vi "MultiLineString_GOOPKernel.vi"(0 "Ref in":i32, 1 "Data in":T4, 2 "Data shared in":T2, 3 "VI ref":string, 4 "Dynamic VI path":path, 5 "Subclass folders":path[](array[path]), 6 "Subclass names":string[](array[string]), 7 "error in (no error)":errorcluster, 8 "Action":T3, 9 "Subclass?":bool, 10 "Object name":string, 11 "Dynamic VI name":string, 13 "First try?":bool, 15 "Occurrence":refnum<k4>, 17 "Occurrence shared":refnum<k4>) -> (14 "Occurrence out":refnum<k4>, 16 "# of objects":i32, 18 "Class statistics":T1, 19 "IsSubclass?":bool, 20 "Ref out":i32, 21 "Data out":T4, 22 "Data shared out":T2, 23 "VI ref out":string, 24 "Dynamic VI path out":path, 25 "Exists?":bool, 26 "Data locked?":bool, 27 "error out":errorcluster)   [LabVIEW 2012, in "MultiLineString.lvclass"]
doc: "This VIs manages objects of the MultiLineString.\n\n[GOOP 2.0.15]"
uses:
  <resource>/Framework/Providers/Open_GDS/UML/MultiLineString_class/MultiLineString.lvclass
  <resource>/Framework/Providers/Open_GDS/UML/MultiLineString_class/protected/ObjectAttributes.ctl
  <resource>/Framework/Providers/Open_GDS/UML/MultiLineString_class/JustificationType.ctl
  <resource>/Framework/Providers/Open_GDS/UML/MultiLineString_class/SizeType.ctl
  <vilib>/addons/_goop3.llb/3GOOPStates.ctl
  <resource>/Framework/Providers/Open_GDS/UML/MultiLineString_class/protected/ClassAttributes.ctl
  <vilib>/addons/_goop3.llb/3GOOPClassStatistics.ctl
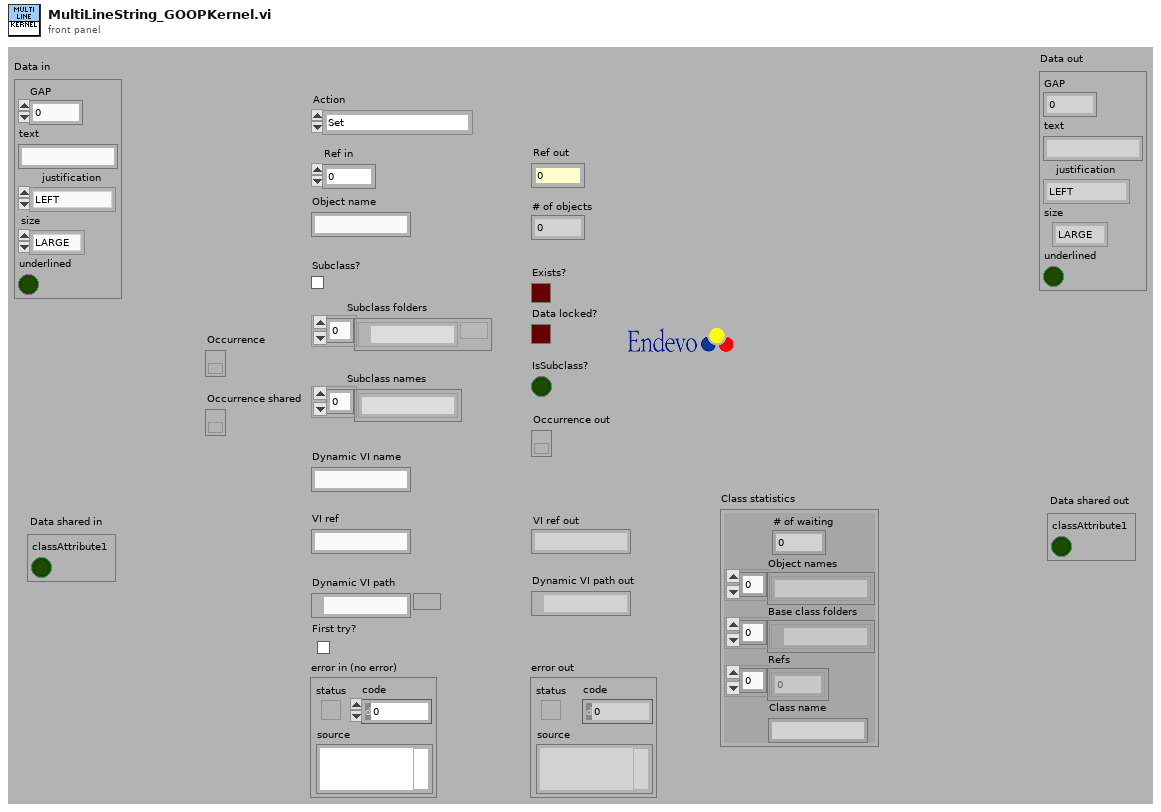
[diagram p1: front panel]
types:
  T1 = typedef "3GOOPClassStatistics.ctl" = cluster{"# of waiting":u32, "Object names":string[], "Base class folders":path[], "Refs":i32[], "Class name":string}
  T2 = typedef "MultiLineString.lvclass/ClassAttributes.ctl" = cluster{"classAttribute1":bool}
  T3 = typedef "3GOOPStates.ctl" = enum16{"Set", "Get", "New", "Delete", "Clear", "Test and get", "Unlock data", "Information", "Look up existing", "New or look up existing", "Test and get shared", "Get shared", "Set shared", "Unlock shared", "Find dynamic method", "Register dynamic method", "Preload dynamic method", "Probe", "Cast to more generic", "Cast to more specific"}
  T4 = typedef "MultiLineString.lvclass/ObjectAttributes.ctl" = cluster{"GAP":i32, "text":string, "justification":T5, "size":T6, "underlined":bool}
  T5 = typedef "MultiLineString.lvclass/JustificationType.ctl" = enum16{"LEFT", "CENTER", "RIGHT"}
  T6 = typedef "MultiLineString.lvclass/SizeType.ctl" = enum16{"LARGE", "NORMAL", "SMALL"}
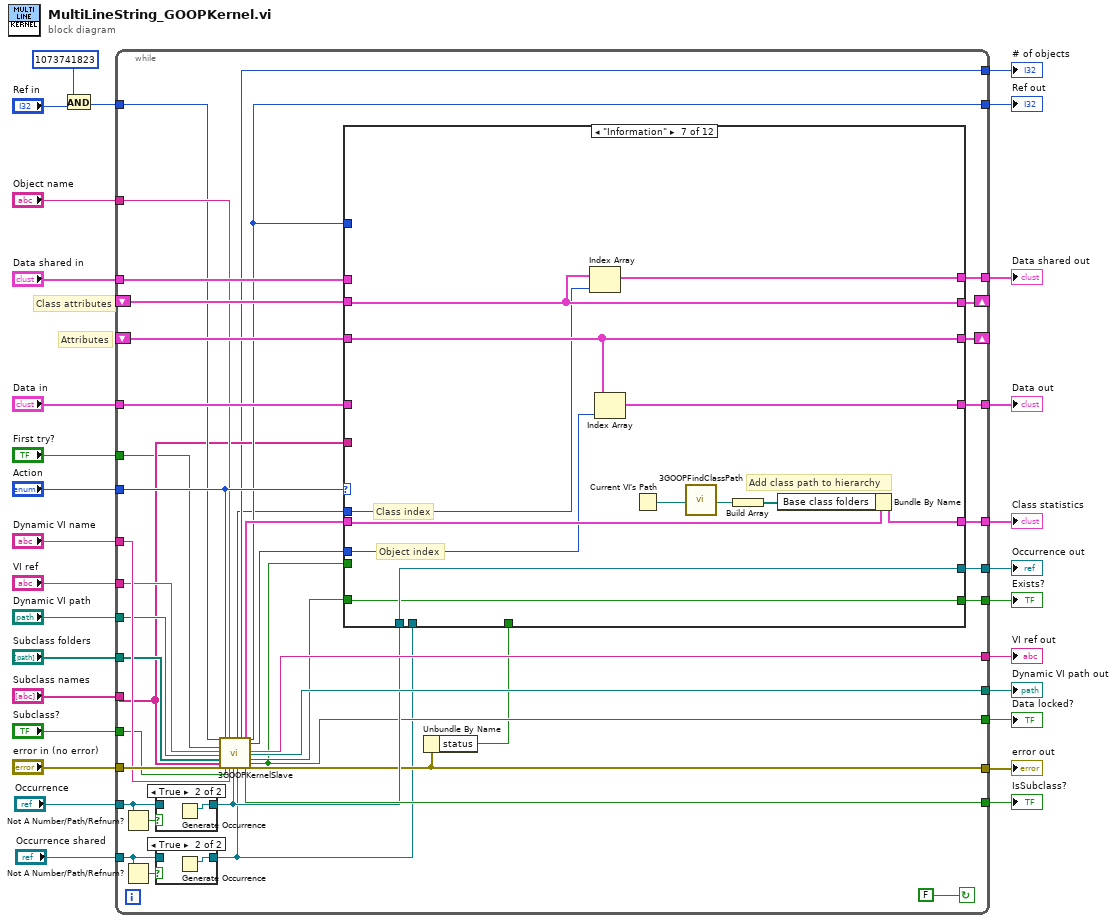
[diagram p0: block diagram]
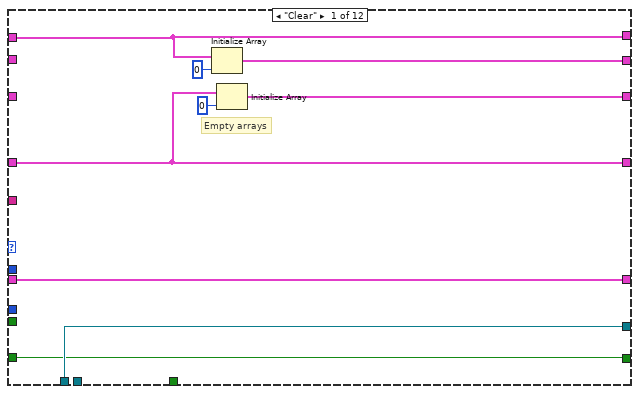
[diagram p4: hidden frame]
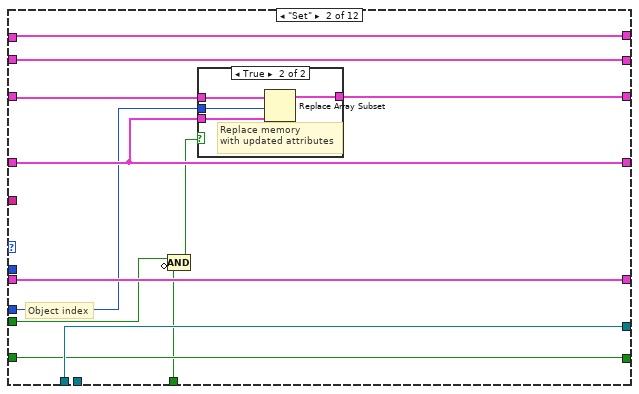
[diagram p5: hidden frame]
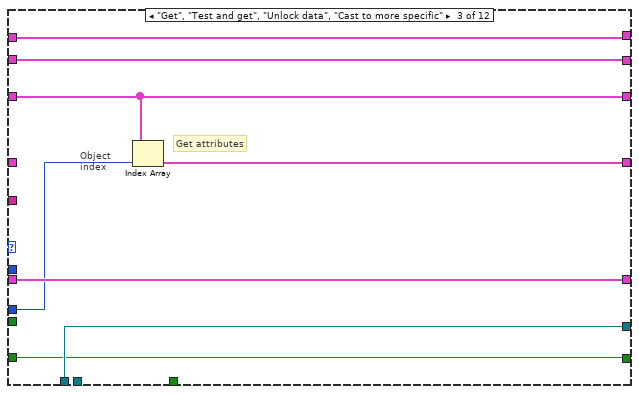
[diagram p7: hidden frame]
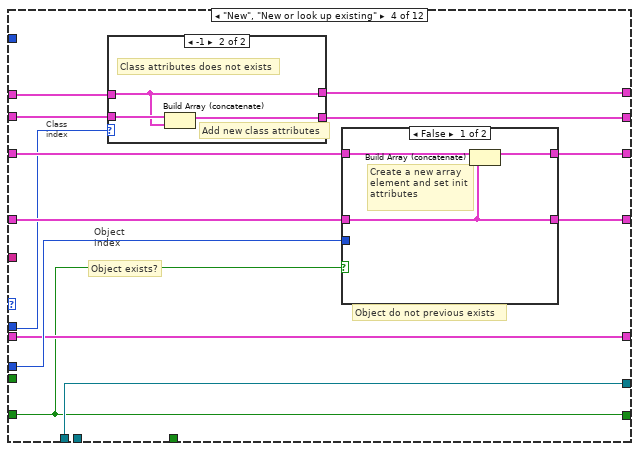
[diagram p8: hidden frame]
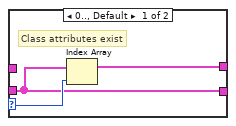
[diagram p9: hidden frame]
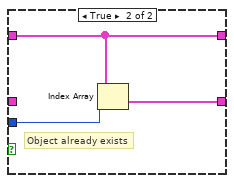
[diagram p10: hidden frame]
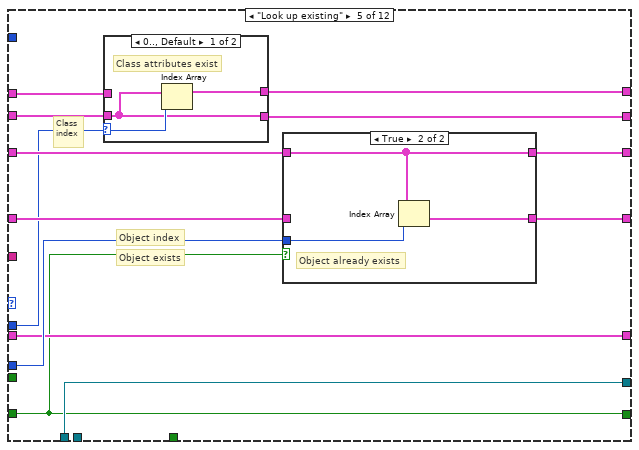
[diagram p11: hidden frame]
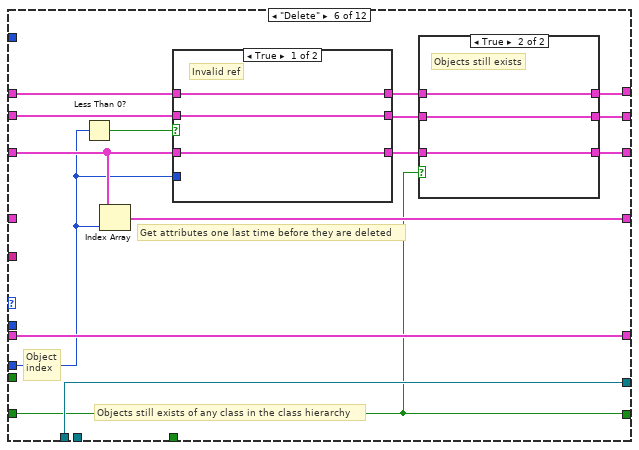
[diagram p14: hidden frame]
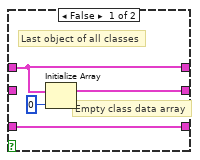
[diagram p15: hidden frame]
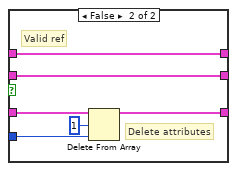
[diagram p16: hidden frame]
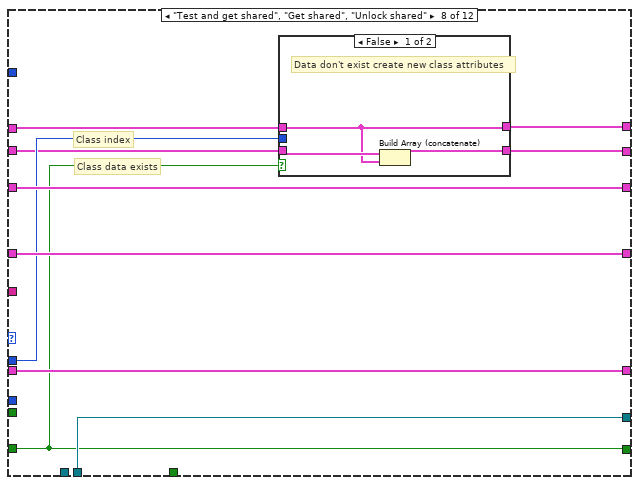
[diagram p17: hidden frame]
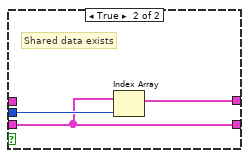
[diagram p18: hidden frame]
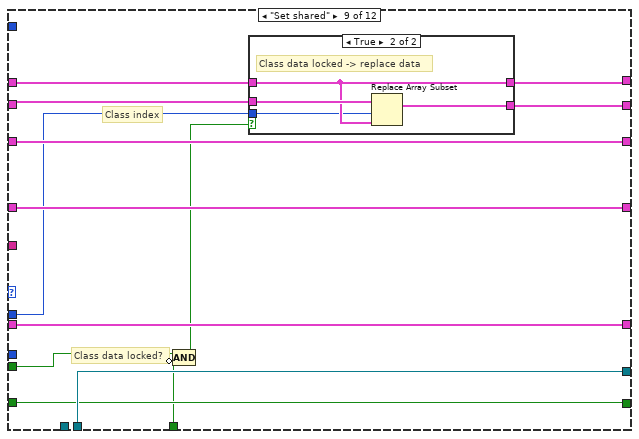
[diagram p19: hidden frame]
diagram:
  # "Attributes"
  # "Class attributes"
  n1 = And(x=1073741823 ("x .and. y?"), y="Ref in") -> (x .and. y?=w3:i32)
  n2 = while {
    tunnel: [w37] -> w6
    tunnel: [w41] -> w7
    tunnel: [w43] -> w8
    tunnel: "First try?" -> [w44]
    tunnel: [w46] -> w10
    tunnel: [w47] -> w11
    tunnel: [w62] -> w13
    tunnel: "Subclass folders" -> [w58]
    tunnel: "Subclass names" -> [w45]
    tunnel: "VI ref" -> [w56]
    tunnel: [w51] -> w17
    tunnel: "Dynamic VI path" -> [w57]
    tunnel: [w50] -> w19
    tunnel: "Dynamic VI name" -> [w60]
    tunnel: "Data shared in" -> [w63]
    shift-left: _ -> [w64]
    shift-right: [w65] -> _
    tunnel: "Object name" -> [w54]
    tunnel: [w36] -> w23
    tunnel: "error in (no error)" -> [w61]
    tunnel: "Subclass?" -> [w59]
    tunnel: [w38] -> w26
    tunnel: [w48] -> w27
    tunnel: w3 -> [w49]
    shift-left: _ -> [w68]
    shift-right: [w69] -> _
    tunnel: [w70] -> w28
    tunnel: "Action" -> [w55]
    tunnel: "Data in" -> [w67]
    tunnel: "Occurrence shared" -> [w33]
    tunnel: "Occurrence" -> [w30]
    stop <- FALSE continue-if-true
    n3 = Not A Number/Path/Refnum?(number/path/refnum=w30) -> (NaN/Path/Refnum?=w31:bool)
    n4 = Not A Number/Path/Refnum?(number/path/refnum=w33) -> (NaN/Path/Refnum?=w34:bool)
    n5 = case shown="True" w31 {
      tunnel: w30 -> [w71 _]
      tunnel: [w71 w72] -> w42
      frame False {
      }
      frame True {
        n6 = Generate Occurrence() -> (w72:refnum<k4>)
      }
    }
    n7 = case shown="True" w34 {
      tunnel: w33 -> [w73 _]
      tunnel: [w73 w74] -> w32
      frame False {
      }
      frame True {
        n8 = Generate Occurrence() -> (w74:refnum<k4>)
      }
    }
    n9 = call <vilib>:"3GOOPKernelSlave.vi"("ref in"=w49, "Misc"=w44, "Probe in"=w56, "Dynamic VI path"=w57, "Subclass folders"=w58, "Subclass names"=w45, "error in (no error)"=w61, "Action"=w55, "Subclass?"=w59, "Object name"=w54, "Class name"=w60, "Occurrence"=w42, "Occurrence shared"=w32) -> ("Shared index out"=w40:i32, "# of objects"=w43:i32, "Class statistics"=w52:T1, "IsSubclass?"=w47:bool, "ref out"=w48:i32, "Index out"=w53:i32, "Probe out"=w50:string, "Dynamic VI path out"=w51:path, "Exists/DynamicCall?"=w39:bool, "Data locked?"=w38:bool, "error out"=w36:errorcluster)  [unwired: 1 in, 3 out]
    n10 = Unbundle By Name(w36) -> ("status"=w35:bool)
    n11 = case shown="\"Information\"" w55 {
      tunnel: [w77 w95 w107 w118 w143 w168 w199 w210 w228 w242 w253 w254] -> w70
      tunnel: [w78 w93 w108 w120 w145 w159 w200 w209 w229 w240 w248 w255] -> w69
      tunnel: w68 -> [_ w94 w108 w121 w146 w171 w200 w209 w229 w240 w248 w255]
      tunnel: w67 -> [w77 w95 _ w119 w144 _ _ w210 w228 w242 w253 w254]
      tunnel: [w80 w92 w106 w112 w136 w162 w193 w201 w225 w241 w249 w259] -> w65
      tunnel: w64 -> [_ w92 w106 w114 w140 w169 w193 w202 w226 w241 w249 w259]
      tunnel: w63 -> [w81 w89 w103 w115 w139 w165 _ w206 w224 w238 w251 w260]
      tunnel: [w83 w91 w105 w116 w141 w167 w197 w208 w227 w239 w252 w258] -> w62
      tunnel: w38 -> [_ w85 _ _ _ _ _ _ w218 _ _ _]
      tunnel: w53 -> [_ w90 w104 w117 w142 w166 w195 _ _ _ _ _]
      tunnel: w52 -> [w83 w91 w105 w116 w141 w167 w196 w208 w227 w239 w252 w258]
      tunnel: w48 -> [_ _ _ _ _ _ _ _ _ _ _ _]
      tunnel: w39 -> [w75 w87 w101 w109 w134 w157 w188 w203 w220 w236 w243 w256]
      tunnel: [w81 w89 w103 w111 w137 w163 w194 w207 w223 w238 w251 w260] -> w46
      tunnel: w45 -> [_ _ _ _ _ _ _ _ _ _ _ _]
      tunnel: w42 -> [w76 w88 w102 w110 w135 w158 w191 _ _ w237 w250 w257]
      tunnel: w32 -> [_ _ _ _ _ _ _ w204 w221 _ _ _]
      tunnel: [w76 w88 w102 w110 w135 w158 w191 w204 w221 w237 w250 w257] -> w41
      tunnel: w40 -> [_ _ _ w113 w138 _ w192 w205 w222 _ _ _]
      tunnel: [w75 w87 w101 w109 w134 w157 w188 w203 w220 w236 w245 w256] -> w37
      tunnel: w35 -> [_ w86 _ _ _ _ _ _ w219 _ _ _]
      frame "Clear" {
        # "Empty arrays"
        n12 = Initialize Array(w81, 0 ("Dimension Size")) -> (w80:T2[])
        n13 = Initialize Array(w77, 0 ("Dimension Size")) -> (w78:T4[])
      }
      frame "Set" {
        # "Object index"
        n14 = Compound Arithmetic op=AND(w85, invert w86) -> (w84:bool)
        n15 = case shown="True" w84 {
          tunnel: w95 -> [_ w100]
          tunnel: w94 -> [w96 w99]
          tunnel: [w96 w98] -> w93
          tunnel: w90 -> [_ w97]
          frame False {
            # "Attributes not locked!"
          }
          frame True {
            # "Replace memory\nwith updated attributes"
            n16 = Replace Array Subset(array=w99, new element=w100, index=w97) -> (w98:T4[])
          }
        }
      }
      frame "Get", "Test and get", "Unlock data", "Cast to more specific" {
        # "Object\nindex"
        # "Get attributes"
        n17 = Index Array(array=w108, index=w104) -> (element=w107:T4)
      }
      frame "New", "New or look up existing" {
        # "Object exists?"
        # "Object\nindex"
        # "Class\nindex"
        n18 = case shown="-1" w113 {
          selector: w113 -> [w124 _]
          tunnel: w115 -> [_ w125]
          tunnel: w114 -> [w123 w127]
          tunnel: [w123 w126] -> w112
          tunnel: [w122 w125] -> w111
          frame 0.., Default {
            # "Class attributes exist"
            n19 = Index Array(array=w123, index=w124) -> (element=w122:T2)
          }
          frame -1 {
            # "Add new class attributes"
            # "Class attributes does not exists"
            n20 = Build Array (concatenate)(w127, w125) -> (w126:T2[])
          }
        }
        n21 = case shown="False" w109 {
          tunnel: w121 -> [w130 w133]
          tunnel: [w129 w133] -> w120
          tunnel: w119 -> [w128 _]
          tunnel: [w128 w132] -> w118
          tunnel: w117 -> [_ w131]
          frame False {
            # "Object do not previous exists"
            # "Create a new array \nelement and set init\nattributes"
            n22 = Build Array (concatenate)(w130, w128) -> (w129:T4[])
          }
          frame True {
            # "Object already exists"
            n23 = Index Array(array=w133, index=w131) -> (element=w132:T4)
          }
        }
      }
      frame "Look up existing" {
        # "Object exists"
        # "Object index"
        # "Class\nindex"
        n24 = case shown="0.., Default" w138 {
          selector: w138 -> [w149 _]
          tunnel: w139 -> [_ w151]
          tunnel: w140 -> [w148 w150]
          tunnel: [w148 w150] -> w136
          tunnel: [w147 w151] -> w137
          frame 0.., Default {
            # "Class attributes exist"
            n25 = Index Array(array=w148, index=w149) -> (element=w147:T2)
          }
          frame -1 {
            # "Class does not exist"
          }
        }
        n26 = case shown="True" w134 {
          tunnel: w146 -> [w153 w155]
          tunnel: [w153 w155] -> w145
          tunnel: w144 -> [w152 _]
          tunnel: [w152 w154] -> w143
          tunnel: w142 -> [_ w156]
          frame False {
            # "Object do not previous exists"
          }
          frame True {
            # "Object already exists"
            n27 = Index Array(array=w155, index=w156) -> (element=w154:T4)
          }
        }
      }
      frame "Delete" {
        # "Objects still exists of any class in the class hierarchy"
        # "Object\nindex"
        # "Get attributes one last time before they are deleted"
        n28 = Less Than 0?(x=w166) -> (x < 0?=w170:bool)
        n29 = Index Array(array=w171, index=w166) -> (element=w168:T4)
        n30 = case shown="True" w170 {
          tunnel: w171 -> [w181 w186]
          tunnel: [w181 w185] -> w160
          tunnel: w166 -> [_ w183]
          tunnel: w169 -> [w180 w184]
          tunnel: [w180 w184] -> w161
          tunnel: w165 -> [w179 w182]
          tunnel: [w179 w182] -> w164
          frame True {
            # "Invalid ref"
          }
          frame False {
            # "Delete attributes"
            # "Valid ref"
            n31 = Delete From Array(array=w186, length=1 ("Length"), index=w183) -> (array with subset deleted=w185:T4[])  [unwired: 1 out]
          }
        }
        n32 = case shown="True" w157 {
          tunnel: w164 -> [w172 w178]
          tunnel: [w172 w178] -> w163
          tunnel: [w173 w177] -> w162
          tunnel: w161 -> [_ w177]
          tunnel: w160 -> [w175 w176]
          tunnel: [w175 w176] -> w159
          frame False {
            # "Empty class data array"
            # "Last object of all classes"
            n33 = Initialize Array(w172, 0 ("Dimension Size")) -> (w173:T2[])
          }
          frame True {
            # "Objects still exists"
          }
        }
      }
      frame "Information" {
        # "Object index"
        # "Class index"
        # "Add class path to hierarchy"
        n34 = Index Array(array=w193, index=w192) -> (element=w194:T2)
        n35 = Index Array(array=w200, index=w195) -> (element=w199:T4)
        n36 = Current VI's Path() -> (path=w198:path)
        n37 = call <vilib>:"3GOOPFindClassPath.vi"("current VI path"=w198) -> ("Class folder"=w189:path)  [unwired: 18 out]
        n38 = Build Array(w189) -> (w190:path[])
        n39 = Bundle By Name(cluster=w196, "Base class folders"=w190) -> (w197:T1)
      }
      frame "Test and get shared", "Get shared", "Unlock shared" {
        # "Class index"
        # "Class data exists"
        n40 = case shown="False" w203 {
          tunnel: [w211 w215] -> w207
          tunnel: w202 -> [w213 w214]
          tunnel: w205 -> [_ w216]
          tunnel: w206 -> [w211 _]
          tunnel: [w212 w214] -> w201
          frame False {
            # "Data don't exist create new class attributes"
            n41 = Build Array (concatenate)(w213, w211) -> (w212:T2[])
          }
          frame True {
            # "Shared data exists"
            n42 = Index Array(array=w214, index=w216) -> (element=w215:T2)
          }
        }
      }
      frame "Set shared" {
        # "Class data locked?"
        # "Class index"
        n43 = Compound Arithmetic op=AND(w218, invert w219) -> (w217:bool)
        n44 = case shown="True" w217 {
          tunnel: w226 -> [w231 w235]
          tunnel: [w231 w234] -> w225
          tunnel: w224 -> [w230 w233]
          tunnel: [w230 w233] -> w223
          tunnel: w222 -> [_ w232]
          frame False {
            # "Shared data not locked -> error do not update"
          }
          frame True {
            # "Class data locked -> replace data"
            n45 = Replace Array Subset(array=w235, new element=w233, index=w232) -> (w234:T2[])
          }
        }
      }
      frame "Find dynamic method".."Preload dynamic method" {
      }
      frame "Probe" {
        # "Any shiftregister array in Kernel Slave has elements?"
        # "Any shiftregister array has elements?"
        # "Check if memory cleared"
        n46 = Array Size(array=w248) -> (size(s)=w247:i32)
        n47 = Equal To 0?(x=w247) -> (x = 0?=w246:bool)
        n48 = Compound Arithmetic op=AND(w246) -> (invert w244:bool)
        n49 = Or(x=w244, y=w243) -> (x .or. y?=w245:bool)
      }
      frame "Cast to more generic", Default {
      }
    }
  }
  "Data out" <- w28
  "Ref out" <- w27
  "Data locked?" <- w26
  "error out" <- w23
  "Exists?" <- w6
  "Data shared out" <- w10
  "VI ref out" <- w19
  "Dynamic VI path out" <- w17
  "Class statistics" <- w13
  "IsSubclass?" <- w11
  "# of objects" <- w8
  "Occurrence out" <- w7
